vi "CalculateCOSHalfTheta.vi"(10 "qb":T1, 11 "qa":T1) -> (0 "cosHalfTheta >= 1":bool, 3 "cosHalfTheta":dbl)   [LabVIEW 2016]
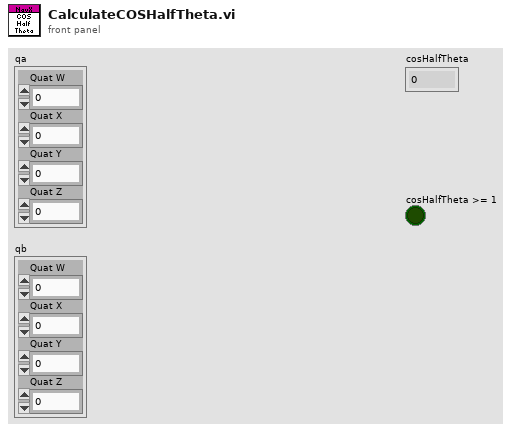
[diagram p1: front panel]
types:
  T1 = cluster{"Quat W":dbl, "Quat X":dbl, "Quat Y":dbl, "Quat Z":dbl}
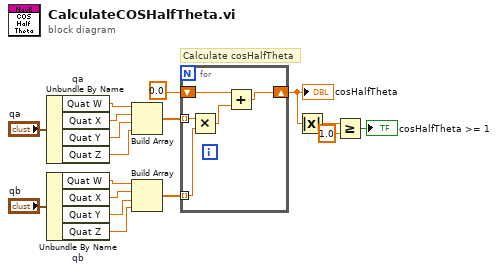
[diagram p0: block diagram]
diagram:
  # "Calculate cosHalfTheta"
  n1 = Unbundle By Name "qa"("qa") -> ("Quat W"=w7:dbl, "Quat X"=w8:dbl, "Quat Y"=w9:dbl, "Quat Z"=w10:dbl)
  n2 = Unbundle By Name "qb"("qb") -> ("Quat W"=w11:dbl, "Quat X"=w12:dbl, "Quat Y"=w13:dbl, "Quat Z"=w14:dbl)
  n3 = Build Array(w7, w8, w9, w10) -> (w15:dbl[])
  n4 = Build Array(w11, w12, w13, w14) -> (w16:dbl[])
  n5 = for {
    tunnel: w15 -> [w22] mode=indexing
    tunnel: w16 -> [w21] mode=indexing
    shift-right: [w18] -> w4
    shift-left: 0.0 -> [w20]
    n6 = Multiply(x=w22, y=w21) -> (x*y=w19:dbl)
    n7 = Add(x=w20, y=w19) -> (x+y=w18:dbl)
  }
  "cosHalfTheta" <- w4
  n8 = Absolute Value(x=w4) -> (abs(x)=w1:dbl)
  n9 = Greater Or Equal?(x=w1, y=1.0) -> (x >= y?=→"cosHalfTheta >= 1":bool)
